vi "Front Camera Circle detect.vi"() -> ()   [LabVIEW 2014]
uses:
  <vilib>/vision/Shape Detection.llb/ShapeDetectionMatchOptions.ctl
  <vilib>/vision/Pattern Matching.llb/IMAQ Match Range Setting.ctl
  <vilib>/vision/Pattern Matching.llb/IMAQ Curve Parameters.ctl
  AR.Drone 2.0 - Phase 4 - Auto hover above object with Video&Navdata method/Global.vi
  <vilib>/vision/NI_Vision_Development_Module.lvlib
panel:
  in  "Circle Index":i32
  out "Score":dbl
  out "Number of Matches Returned":i32
  in  "Curve Parameters":T1={"Extraction Mode"=0, "Edge Threshold"=150, "Edge Filter Size"=1, "Min Length"=25, "Row Search Step Size"=15, "Col Search Step Size"=15, "Max Endpoint Gap"=10, "Closed"=TRUE, "Subpixel"=FALSE} {"Extraction Mode" items=["Normal", "Uniform Regions"]; "Edge Filter Size" items=["Fine", "Normal", "Contour Tracing"]; "Max Endpoint Gap" min=0; "Col Search Step Size" min=1 max=255 step=1; "Row Search Step Size" min=1 max=255 step=1; "Min Length" min=0; "Edge Threshold" min=1 max=350 step=1}
  out "error out":errorcluster
  in  "Minimum match score":dbl=900.0
  in  "Match Options":T2={"Rotation"=FALSE, "Scale"=FALSE, "Occlusion"=TRUE, "Range Settings"=[{"Match Constraints"=0, "Min"=0.0, "Max"=0.0}, {"Match Constraints"=1, "Min"=0.0, "Max"=0.0}, {"Match Constraints"=2, "Min"=0.0, "Max"=25.0}]} {"Range Settings"."Max" format="%.2f"; "Range Settings"."Min" format="%.2f"; "Range Settings"."Match Constraints" items=["Rotation Angle (degrees)", "Scale Factor (%)", "Occlusion (%)"]}
  in  "Circle Descriptor":cluster{"Min Radius":dbl, "Max Radius":dbl}={"Min Radius"=20.0, "Max Radius"=400.0}
  out "Image":T4(plugin-control)
  in  "milliseconds to wait":u32
  out "Read Video":errorcluster
  out "x-y":u32=19
  # "Range"
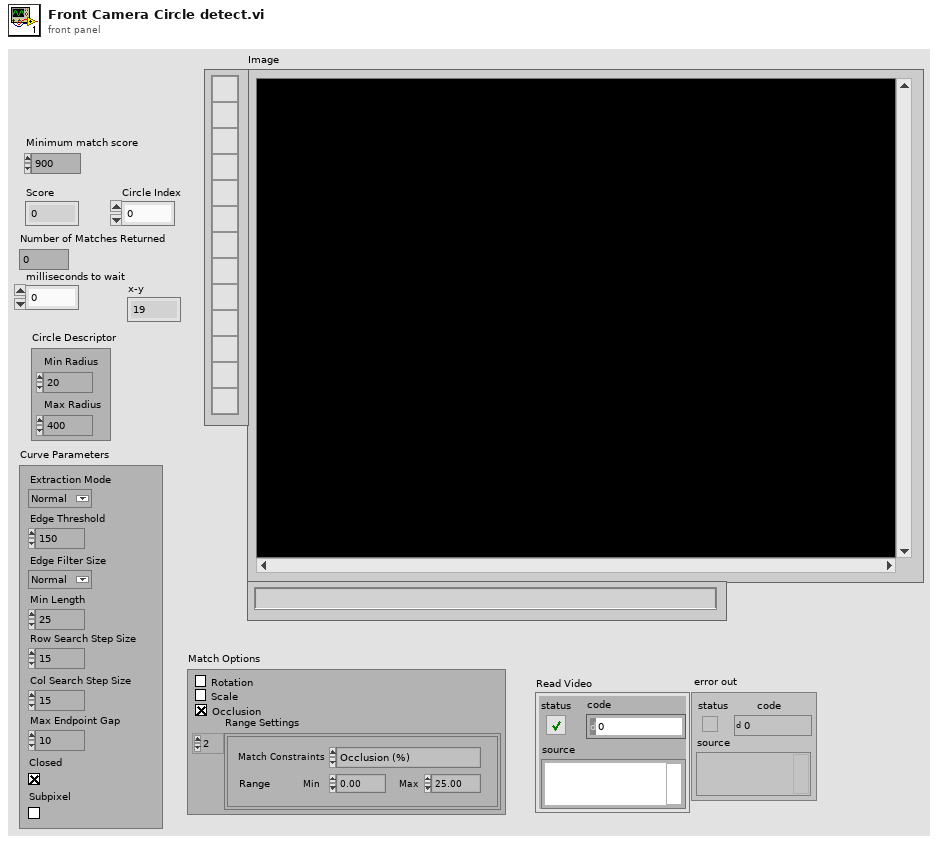
[diagram p1: front panel]
types:
  T1 = typedef "IMAQ Curve Parameters.ctl" = cluster{"Extraction Mode":u32, "Edge Threshold":i32, "Edge Filter Size":u32, "Min Length":i32, "Row Search Step Size":i32, "Col Search Step Size":i32, "Max Endpoint Gap":i32, "Closed":bool, "Subpixel":bool}
  T2 = typedef "ShapeDetectionMatchOptions.ctl" = cluster{"Rotation":bool, "Scale":bool, "Occlusion":bool, "Range Settings":T3[]}
  T3 = typedef "IMAQ Match Range Setting.ctl" = cluster{"Match Constraints":u32, "Min":dbl, "Max":dbl}
  T4 = typedef "IMAQ Image.ctl" = refnum<image>
  T5 = typedef "Image Type" = u32
  T6 = cluster{"Position":cluster{"X":sgl, "Y":sgl}, "Radius":dbl, "Score":dbl}[]
  T7 = cluster{"Position":cluster{"X":sgl, "Y":sgl}, "Radius":dbl, "Score":dbl}
  T8 = cluster{"Left":i32, "Top":i32, "Right":i32, "Bottom":i32}
  T9 = typedef "Control cluster.ctl" = cluster{"Roll":sgl, "Pitch":sgl, "Vertical Speed":sgl, "Yaw Speed":sgl}
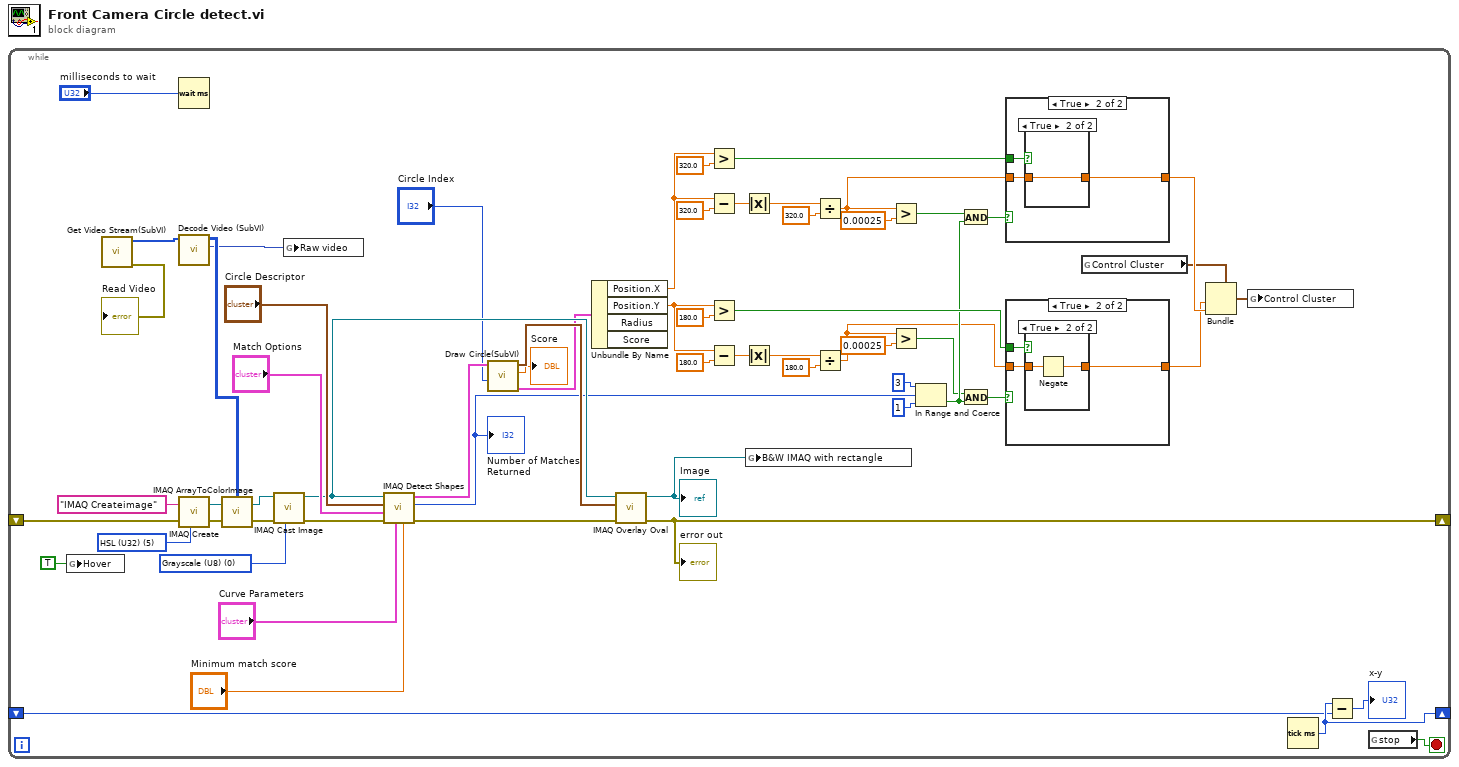
[diagram p0: block diagram]
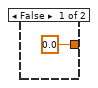
[diagram p2: hidden frame]
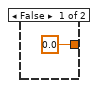
[diagram p4: hidden frame]
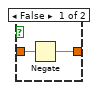
[diagram p5: hidden frame]
diagram:
  n1 = while {
    shift-right: [w54] -> _
    shift-left: _ -> [w53]
    shift-right: [w39] -> _
    shift-left: _ -> [w50]
    stop <- w8 stop-if-true
    w47 = T5 0 items=["Grayscale (U8)", "Grayscale (I16)", "Grayscale (SGL)", "Complex (CSG)", "RGB (U32)", "HSL (U32)", "RGB (U64)", "Grayscale (U16)"] ("Image Type")
    w60 = T5 5 items=["Grayscale (U8)", "Grayscale (I16)", "Grayscale (SGL)", "Complex (CSG)", "RGB (U32)", "HSL (U32)", "RGB (U64)", "Grayscale (U16)"] ("Image Type")
    n2 = global write "Global.vi" "Hover"(TRUE) -> ()
    n3 = call "Get Video Stream(SubVI).vi"() -> ("error out"=→"Read Video":errorcluster, "ImgData"=w61:u8[])  [unwired: 10 in]
    n4 = Wait (ms)(milliseconds to wait="milliseconds to wait") -> ()  [unwired: 1 out]
    n5 = call "Decode Video (SubVI).vi"("ImgData"=w61) -> ("new picture"=w51:picture, "Array"=w57:u32[][])  [unwired: 9 in]
    n6 = call "IMAQ Create"("Image Name"="IMAQ Createimage", "Image Type"=w60, "error in (no error)"=w50) -> ("New Image"=w56:T4, "error out"=w55:errorcluster)  [unwired: 2 in]
    n7 = call "IMAQ ArrayToColorImage"("Image Pixels (U32)"=w57, "Image"=w56, "error in (no error)"=w55) -> ("Image Out"=w48:T4, "error out"=w49:errorcluster)  [unwired: 2 in]
    n8 = call "IMAQ Cast Image"("Image Type"=w47, "error in (no error)"=w49, "Image Src"=w48) -> ("error out"=w44:errorcluster, "Image Dst Out"=w42:T4)  [unwired: 7 in]
    n9 = global write "Global.vi" "Raw video"(w51) -> ()
    n10 = call-poly "IMAQ Detect Shapes"("Minimum match score"="Minimum match score", "Curve Parameters"="Curve Parameters", "error in (no error)"=w44, "Match Options"="Match Options", "Circle Descriptor"="Circle Descriptor", "Image"=w42) -> ("error out"=w41:errorcluster, "Number of Matches Returned"=w11:i32, "Circles"=w37:T6)  [unwired: 3 in]
    "Number of Matches Returned" <- w11
    n11 = call "Draw Circle(SubVI).vi"("Circle Index"="Circle Index", "Circles"=w37) -> ("element"=w35:T7, "Score"=→"Score":dbl, "Bounding Rectangle out"=w40:T8)  [unwired: 7 in]
    n12 = Unbundle By Name(w35) -> ("Position.X"=w20:sgl, "Position.Y"=w25:sgl)  [unwired: 2 out]
    n13 = call "IMAQ Overlay Oval"("error in (no error)"=w41, "Bounding Rectangle"=w40, "Image"=w42) -> ("error out"=w39:errorcluster, "Image Out"=w33:T4)  [unwired: 7 in]
    "Image" <- w33
    "error out" <- w39
    n14 = Greater?(x=w20, y=320.0) -> (0:w18:bool)
    n15 = Subtract(x=w20, y=320.0) -> (x-y=w23:dbl)
    n16 = Greater?(x=w25, y=180.0) -> (0:w31:bool)
    n17 = Subtract(x=w25, y=180.0) -> (x-y=w28:dbl)
    n18 = Absolute Value(x=w23) -> (abs(x)=w22:dbl)
    n19 = Absolute Value(x=w28) -> (abs(x)=w27:dbl)
    n20 = global write "Global.vi" "B&W IMAQ with rectangle"(w33) -> ()
    n21 = Divide(x=w22, y=320.0) -> (x/y=w16:dbl)
    n22 = Divide(x=w27, y=180.0) -> (x/y=w3:dbl)
    n23 = Greater?(x=w16, y=0.00025) -> (0:w13:bool)
    n24 = Greater?(x=w3, y=0.00025) -> (0:w1:bool)
    n25 = In Range and Coerce(upper limit=3, x=w11, lower limit=1) -> (In Range?=w4:bool)  [unwired: 1 out]
    n26 = And(x=w13, y=w4) -> (x .and. y?=w14:bool)
    n27 = And(x=w1, y=w4) -> (x .and. y?=w5:bool)
    n28 = case shown="True" w14 {
      tunnel: w18 -> [_ w73]
      tunnel: [0.0 w72] -> w17
      tunnel: w16 -> [_ w71]
      frame False {
      }
      frame True {
        n29 = case shown="True" w73 {
          tunnel: w71 -> [w75 w76]
          tunnel: [w74 w76] -> w72
          frame False {
            n30 = Negate(x=w75) -> (-x=w74:dbl)
          }
          frame True {
          }
        }
      }
    }
    n31 = case shown="True" w5 {
      tunnel: w31 -> [_ w66]
      tunnel: w3 -> [_ w65]
      tunnel: [0.0 w64] -> w6
      frame False {
      }
      frame True {
        n32 = case shown="True" w66 {
          tunnel: w65 -> [w67 w69]
          tunnel: [w67 w68] -> w64
          frame False {
          }
          frame True {
            n33 = Negate(x=w69) -> (-x=w68:dbl)
          }
        }
      }
    }
    n34 = global read "Global.vi" "Control Cluster"() -> (w7:T9)
    n35 = Bundle(cluster=w7, "Vertical Speed"=w6, "Yaw Speed"=w17) -> (w34:T9)  [unwired: 2 in]
    n36 = global write "Global.vi" "Control Cluster"(w34) -> ()
    n37 = Tick Count (ms)() -> (millisecond timer value=w54:u32)
    n38 = Subtract(x=w54, y=w53) -> (x-y=→"x-y":u32)
    n39 = global read "Global.vi" "stop"() -> (w8:bool)
  }
